vi "Update Experiment_Experimenter_Sample details in DOM Object.vi"(8 "error in (no error)":errorcluster, 10 "Experiment|_Experimenter_Sample_Cluster IN":T1, 11 "Refnum in":refnum<k20>) -> (0 "error out":errorcluster)   [LabVIEW 2012]
doc: "SciScan 1.2 160622"
uses:
  Custom Controls and Typedefs/Experiment and Experimenter.ctl
  <vilib>/xml/NI_XML.lvlib
  <resource>/objmgr/DOMUserDefRef.rc
panel:
  # "Experiment"
  # "Experimenter"
  # "Sample"
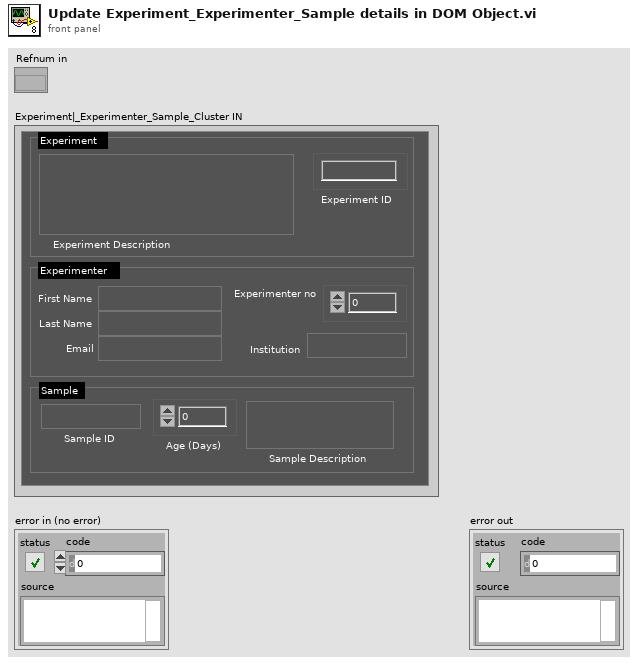
[diagram p1: front panel]
types:
  T1 = typedef "Experiment and Experimenter.ctl" = cluster{"Experimenter no":u32, "First Name":string, "Experiment ID":string, "urn:lsid: ":string, "Experiment Description":string, "Last Name":string, "Email":string, "Institution":string, "Sample ID":string, "Age (Days)":u32, "Sample Description":string}
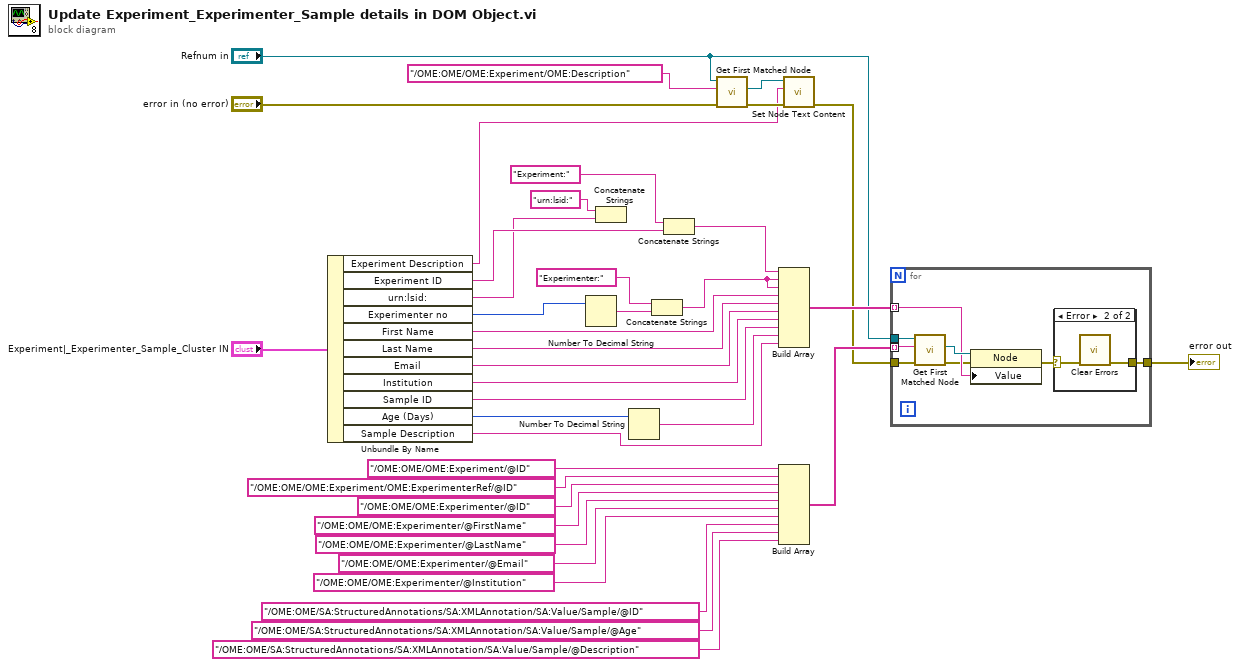
[diagram p0: block diagram]
diagram:
  n1 = Unbundle By Name("Experiment|_Experimenter_Sample_Cluster IN") -> ("Experiment Description"=w4:string, "Experiment ID"=w12:string, "urn:lsid:"=w11:string, "Experimenter no"=w14:u32, "First Name"=w25:string, "Last Name"=w26:string, "Email"=w27:string, "Institution"=w29:string, "Sample ID"=w30:string, "Age (Days)"=w15:u32, "Sample Description"=w32:string)
  n2 = Number To Decimal String(number=w14) -> (decimal integer string=w13:string)  [unwired: 1 in]
  n3 = Concatenate Strings("urn:lsid:" ("urn:lsid:"), w11) -> ()  [unwired: 1 out]
  n4 = Number To Decimal String(number=w15) -> (decimal integer string=w31:string)  [unwired: 1 in]
  n5 = Concatenate Strings("Experimenter:" ("urn:lsid:"), w13) -> (w36:string)
  n6 = Concatenate Strings("Experiment:" ("urn:lsid:"), w12) -> (w24:string)
  n7 = call <vilib>:"Get First Matched Node.vi"("error in (no error)"="error in (no error)", "XPath expression"="/OME:OME/OME:Experiment/OME:Description" ("urn:lsid:"), "node in"="Refnum in") -> ("error out"=w7:errorcluster, "node result"=w8:refnum<k20>)  [unwired: 6 in, 1 out]
  n8 = Build Array(w24, w36, w36, w25, w26, w27, w29, w30, w31, w32) -> (w34:string[])
  n9 = Build Array("/OME:OME/OME:Experiment/@ID" ("urn:lsid:"), "/OME:OME/OME:Experiment/OME:ExperimenterRef/@ID" ("urn:lsid:"), "/OME:OME/OME:Experimenter/@ID" ("urn:lsid:"), "/OME:OME/OME:Experimenter/@FirstName" ("urn:lsid:"), "/OME:OME/OME:Experimenter/@LastName" ("urn:lsid:"), "/OME:OME/OME:Experimenter/@Email" ("urn:lsid:"), "/OME:OME/OME:Experimenter/@Institution" ("urn:lsid:"), "/OME:OME/SA:StructuredAnnotations/SA:XMLAnnotation/SA:Value/Sample/@ID" ("search string/char (-)"), "/OME:OME/SA:StructuredAnnotations/SA:XMLAnnotation/SA:Value/Sample/@Age" ("search string/char (-)"), "/OME:OME/SA:StructuredAnnotations/SA:XMLAnnotation/SA:Value/Sample/@Description" ("search string/char (-)")) -> (w33:string[])
  n10 = call "Set Node Text Content.vi"("error in (no error)"=w7, "newValue"=w4, "node in"=w8) -> ("error out"=w2:errorcluster)  [unwired: 6 in, 2 out]
  n11 = for {
    tunnel: "Refnum in" -> [w45]
    tunnel: w33 -> [w44] mode=indexing
    tunnel: w34 -> [w43] mode=indexing
    tunnel: [w41] -> w35
    tunnel: w2 -> [w40]
    n12 = call <vilib>:"Get First Matched Node.vi"("error in (no error)"=w40, "XPath expression"=w44, "node in"=w45) -> ("error out"=w39:errorcluster, "node result"=w46:refnum<k20>)  [unwired: 6 in, 1 out]
    n13 = property class="Node"(reference=w46, error in=w39, "Value"=w43) -> (error out=w42:errorcluster)  [unwired: 1 out]
    n14 = case shown="Error" w42 {
      selector: w42 -> [w47 w49]
      tunnel: [w47 w48] -> w41
      frame No Error {
      }
      frame Error {
        n15 = call <vilib>:"Clear Errors.vi"("error in (no error)"=w49) -> ("error out"=w48:errorcluster)  [unwired: 6 in]
      }
    }
  }
  "error out" <- w35
